vi "Parse-Incoming-Packet.vi"(11 "Array":u32[](array[numeric]) format="%.0x") -> (1 "Payload (string)":string, 2 "Payload (u8)":u8[](array[numeric]), 3 "Target Session":u8)   [LabVIEW 2018]
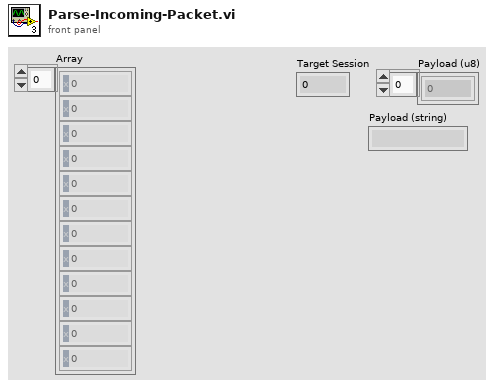
[diagram p1: front panel]
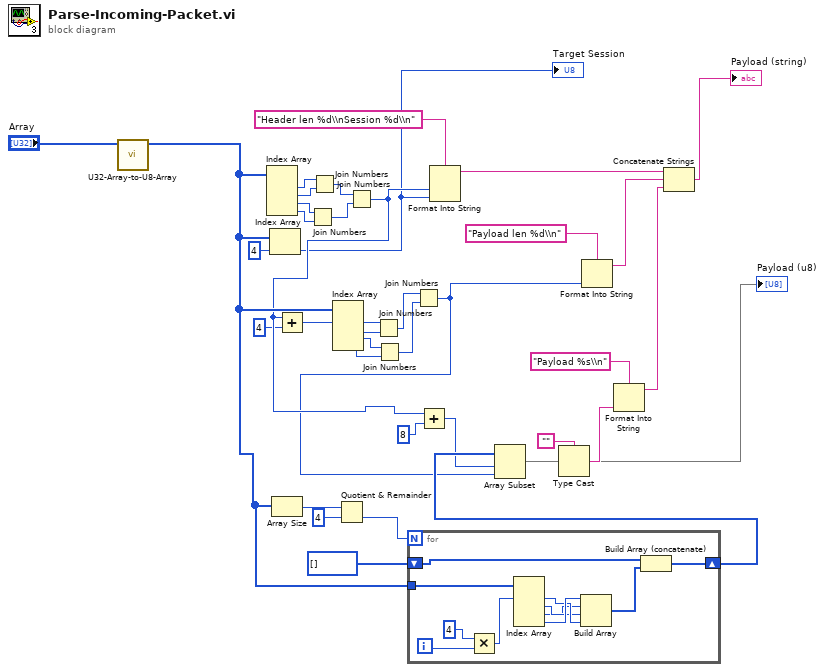
[diagram p0: block diagram]
diagram:
  n1 = call "U32-Array-to-U8-Array.vi"("U32 [] in"="Array") -> ("U8 [] out"=w37:u8[])  [unwired: 10 in]
  n2 = Index Array(array=w37) -> (element #1=w14:u8, element #2=w15:u8, element #3=w13:u8, element #4=w12:u8)  [unwired: 4 in]
  n3 = Index Array(array=w37, index=4) -> (element=w19:u8)
  "Target Session" <- w19
  n4 = Array Size(array=w37) -> (size(s)=w31:i32)
  n5 = Join Numbers(hi=w13, lo=w12) -> ((hi.lo)=w17:u16)
  n6 = Join Numbers(hi=w14, lo=w15) -> ((hi.lo)=w16:u16)
  n7 = Quotient & Remainder(x=w31, y=4) -> (floor(x/y)=w33:i32)  [unwired: 1 out]
  n8 = Join Numbers(hi=w16, lo=w17) -> ((hi.lo)=w36:u32)
  n9 = Add(x=w36, y=u32 4) -> (x+y=w20:u32)
  n10 = Index Array(array=w37, index #1=w20) -> (element #1=w4:u8, element #2=w5:u8, element #3=w22:u8, element #4=w23:u8)  [unwired: 3 in]
  n11 = Join Numbers(hi=w4, lo=w5) -> ((hi.lo)=w24:u16)
  n12 = Join Numbers(hi=w22, lo=w23) -> ((hi.lo)=w25:u16)
  n13 = for {
    N: w33 -> [_]
    tunnel: w37 -> [w48]
    shift-right: [w43] -> w35
    shift-left: u8[] [] -> [w44]
    i -> [w47]
    n14 = Multiply(x=4, y=w47) -> (x*y=w46:i32)
    n15 = Index Array(array=w48, index #1=w46) -> (element #1=w41:u8, element #2=w40:u8, element #3=w39:u8, element #4=w42:u8)  [unwired: 3 in]
    n16 = Build Array(w42, w39, w40, w41) -> (w38:u8[])
    n17 = Build Array (concatenate)(w44, w38) -> (w43:u8[])
  }
  n18 = Join Numbers(hi=w24, lo=w25) -> ((hi.lo)=w30:u32)
  n19 = Add(x=w36, y=u16 8) -> (x+y=w11:u32)
  n20 = Format Into String(format string="Header len %d\\nSession %d\\n", w36, w19) -> (resulting string=w8:string)  [unwired: 2 in, 1 out]
  n21 = Array Subset(array=w35, index=w11, length=w30) -> (w6:u8[])
  "Payload (u8)" <- w6
  n22 = Type Cast(type="", x=w6) -> (*(type *) &x=w28:string)
  n23 = Format Into String(format string="Payload len %d\\n", w30) -> (resulting string=w9:string)  [unwired: 2 in, 1 out]
  n24 = Format Into String(format string="Payload %s\\n", w28) -> (resulting string=w27:string)  [unwired: 2 in, 1 out]
  n25 = Concatenate Strings(w8, w9, w27) -> (→"Payload (string)":string)
